vi "Send Acknowledge Itetations End.vi"(7 "Priority":T1=enum."Normal" caption="Message Priority (Normal)", 8 "error in (no error)":errorcluster, 11 "Message Enqueuer in":refnum<class "Message Enqueuer.lvclass">) -> (0 "error out":errorcluster, 3 "Message Enqueuer out":refnum<class "Message Enqueuer.lvclass">)   [LabVIEW 2023, in "Iterator Actor.lvlib" / "Acknowledge Itetations End Msg.lvclass"]
doc: "Sends the <b>Iterator Actor.lvlib:Acknowledge Itetations End Msg.lvclass</b> message.\n\nThis message will call <b>Acknowledge Itetations End.vi</b> on the <b>Iterator Actor.lvlib:Abstract Iterator Actor.lvclass</b> actor.\n\n<b>Acknowledge Itetations End.vi Description</b>"
uses:
  Acknowledge Itetations End Msg.lvclass
  Acknowledge Itetations End Msg.lvclass/Acknowledge Itetations End Msg.ctl
  <vilib>/ActorFramework/Message Enqueuer/Message Enqueuer.lvclass
  C:/Program Files/National Instruments/LabVIEW 2023/vi.lib/ActorFramework/Message/Message.lvclass
  C:/Projects/Iterator Actor/Abstract Iterator Actor Messages/Acknowledge Itetations End Msg/Acknowledge Itetations End Msg.lvclass
  <vilib>/ActorFramework/Message Enqueuer/Message Priority.ctl
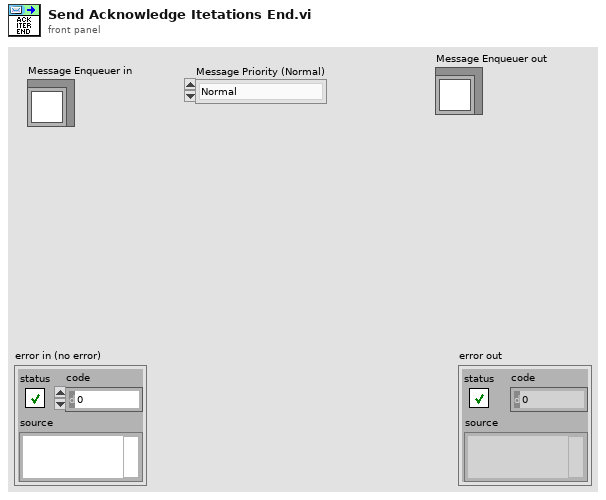
[diagram p1: front panel]
types:
  T1 = typedef "Actor Framework.lvlib/Message Enqueuer.lvclass/Message Priority.ctl" = enum16{"Low", "Normal", "High"}
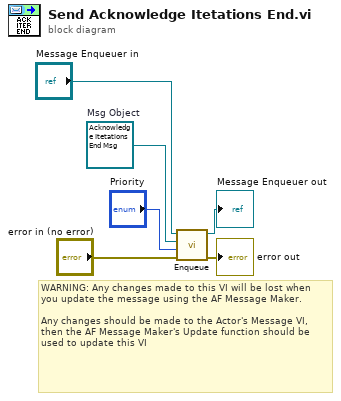
[diagram p0: block diagram]
diagram:
  w2 = refnum<class "Acknowledge Itetations End Msg.lvclass"> refnum  # Msg Object
  # "WARNING: Any changes made to this VI will be lost when you update the message using the AF Message Maker.\n\nAny changes should be made to the Actor's Message VI, then the AF Message Maker's Update function should be used to update this VI"
  n1 = call <vilib>:"Enqueue.vi"("error in (no error)"="error in (no error)", "Message Priority (Normal)"="Priority", "Message"=w2, "Message Enqueuer in"="Message Enqueuer in") -> ("error out"=→"error out":errorcluster, "Message Enqueuer out"=→"Message Enqueuer out":refnum<class "Message Enqueuer.lvclass">)  [unwired: 6 in]
